vi "Read DSF Version.vi"(8 "error in (no error)":errorcluster, 11 "refnum":T2) -> (0 "error out":errorcluster, 2 "dsfversion":T1, 3 "refnum out":T2)   [LabVIEW 2017, in "DSF Configuration API.lvlib"]
doc: "Reads a value associated with a key in a specified section from the configuration data identified by <B>refnum</B>. If the key does not exist, the VI returns the default value. This VI supports multibyte characters in strings. Wire data to the <B>default value</B> input to determine the polymorphic instance to use or manually select the instance."
uses:
  DSF Configuration API.lvlib
  Controls/DSF Config Data RefNum.ctl
  Controls/Version Info.ctl
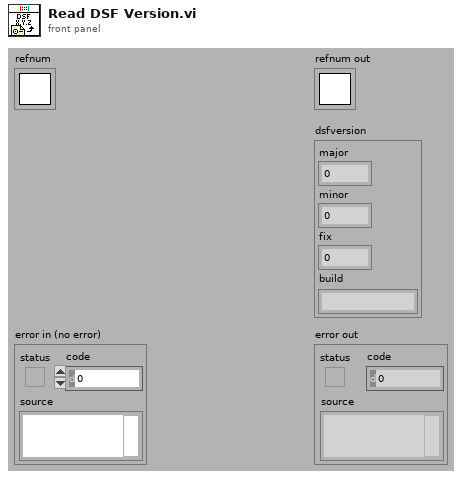
[diagram p1: front panel]
types:
  T1 = typedef "DSF Configuration API.lvlib/Version Info.ctl" = cluster{"major":u32, "minor":u32, "fix":u32, "build":string}
  T2 = typedef "DSF Configuration API.lvlib/DSF Config Data RefNum.ctl" = refnum<k1>
  T3 = typedef "DSF Configuration API.lvlib/Config Queue.ctl" = refnum<queue>
  T4 = typedef "DSF Configuration API.lvlib/Config Data.ctl" = cluster{"dsf configuration":T5, "path":path, "dirty":bool}
  T5 = typedef "DSF Configuration API.lvlib/DSF Config.ctl" = cluster{"dsfversion":T1, "version":T1, "plugins":T6[], "groups":T9[], "transfers":T11[], "channels":T13[], "settings":T15[]}
  T6 = typedef "DSF Configuration API.lvlib/DSF Plugin.ctl" = cluster{"id":string, "values":T7}
  T7 = typedef "DSF Configuration API.lvlib/DSF Plugin Info.ctl" = cluster{"type":string, "timing":T8, "group ids":string[], "settings id":string}
  T8 = typedef "DSF Configuration API.lvlib/DSF Timing Info.ctl" = cluster{"decimation":i32, "offset":i32}
  T9 = typedef "DSF Configuration API.lvlib/DSF Group.ctl" = cluster{"id":string, "values":T10}
  T10 = typedef "DSF Configuration API.lvlib/DSF Group Info.ctl" = cluster{"direction":i32, "timing":T8, "transfer ids":string[], "settings id":string}
  T11 = typedef "DSF Configuration API.lvlib/DSF Transfer.ctl" = cluster{"id":string, "values":T12}
  T12 = typedef "DSF Configuration API.lvlib/DSF Transfer Info.ctl" = cluster{"byte order":i32, "channel ids":string[], "settings id":string}
  T13 = typedef "DSF Configuration API.lvlib/DSF Channel.ctl" = cluster{"id":string, "values":T14}
  T14 = typedef "DSF Configuration API.lvlib/DSF Channel Info.ctl" = cluster{"count":i32, "offset":i32, "data type":i32, "resource path":string, "settings id":string}
  T15 = typedef "DSF Configuration API.lvlib/DSF Settings.ctl" = cluster{"id":string, "values":T16}
  T16 = typedef "DSF Configuration API.lvlib/DSF Settings Info.ctl" = cluster{"key":string, "value":string}[]
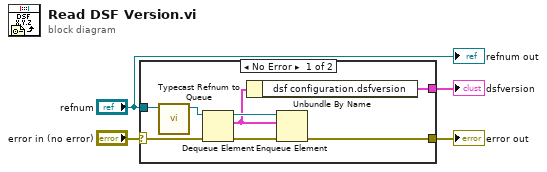
[diagram p0: block diagram]
diagram:
  n1 = case shown="No Error" "error in (no error)" {
    selector: "error in (no error)" -> [w12 w13]
    tunnel: "refnum" -> [w11 _]
    tunnel: [w7 w13] -> w2
    tunnel: [w5 _] -> w1
    frame No Error {
      n2 = call "Typecast Refnum to Queue.vi"("refnum in"=w11) -> ("queue out"=w10:T3)  [unwired: 10 in]
      n3 = Dequeue Element(queue=w10, error in (no error)=w12) -> (queue out=w8:T3, element=w6:T4, error out=w9:errorcluster)  [unwired: 1 in, 1 out]
      n4 = Unbundle By Name(w6) -> ("dsf configuration.dsfversion"=w5:T1)
      n5 = Enqueue Element(queue=w8, element=w6, error in (no error)=w9) -> (error out=w7:errorcluster)  [unwired: 1 in, 2 out]
    }
    frame Error {
    }
  }
  "error out" <- w2
  "dsfversion" <- w1
  "refnum out" <- "refnum"
